vi "NewGrphWindow.vi"(8 "error in (no error)":errorcluster caption="entrée d'erreur (pas d'erreur)", 10 "CurvesIndx":i32[](array[numeric]), 11 "Interface en entrée":refnum<class "Interface.lvclass"> caption="DNL_LabVIEW Object in") -> (0 "error out":errorcluster caption="sortie d'erreur", 3 "Interface en sortie":refnum<class "Interface.lvclass"> caption="DNL_LabVIEW Object out")   [LabVIEW 2010, in "Interface.lvclass"]
uses:
  Interface.lvclass
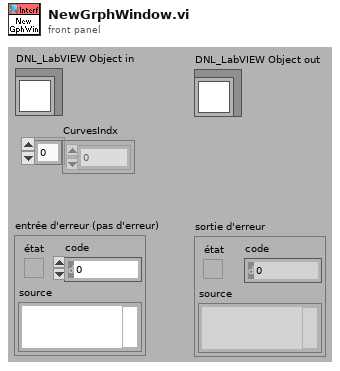
[diagram p1: front panel]
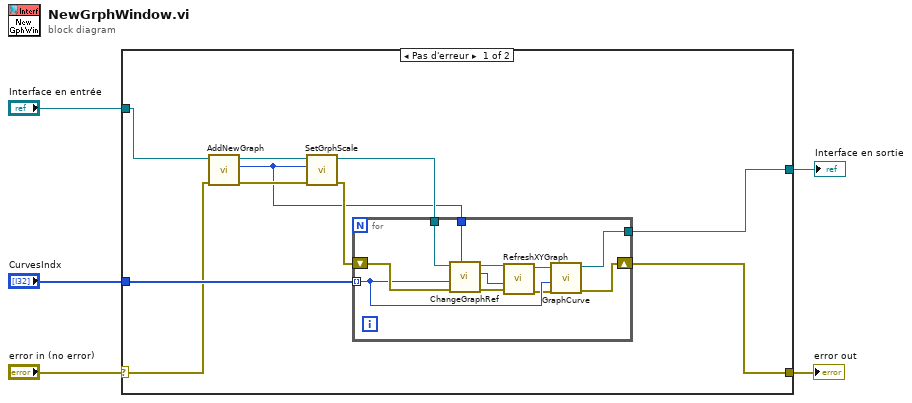
[diagram p0: block diagram]
diagram:
  n1 = case shown="Pas d'erreur" "error in (no error)" {
    selector: "error in (no error)" -> [w12 w28]
    tunnel: [w14 w28] -> w4
    tunnel: [w13 w27] -> w2
    tunnel: "Interface en entrée" -> [w11 w27]
    tunnel: "CurvesIndx" -> [w15 _]
    frame No Error {
      n2 = call "AddNewGraph.vi"("error in (no error)"=w12, "Interface en entrée"=w11) -> ("error out"=w8:errorcluster, "NewGraphInd"=w6:i32, "Interface en sortie"=w10:refnum<class "Interface.lvclass">)  [unwired: 7 in]
      n3 = call "SetGrphScale.vi"("error in (no error)"=w8, "GraphIndex"=w6, "Interface en entrée"=w10) -> ("error out"=w7:errorcluster, "Interface en sortie"=w9:refnum<class "Interface.lvclass">)  [unwired: 7 in]
      n4 = for {
        tunnel: w15 -> [w21] mode=indexing
        tunnel: w9 -> [w25]
        shift-right: [w24] -> w14
        shift-left: w7 -> [w26]
        tunnel: [w23] -> w13
        tunnel: w6 -> [w22]
        n5 = call "ChangeGraphRef.vi"("NewGraphIndex"=w22, "error in (no error)"=w26, "CurveIndex"=w21, "Interface en entrée"=w25) -> ("error out"=w17:errorcluster, "OldGraphIndex"=w16:i32, "Interface en sortie"=w18:refnum<class "Interface.lvclass">)  [unwired: 5 in]
        n6 = call "RefreshXYGraph.vi"("error in (no error)"=w17, "Graph Index"=w16, "Interface en entrée"=w18) -> ("error out"=w20:errorcluster, "Interface en sortie"=w19:refnum<class "Interface.lvclass">)  [unwired: 5 in, 2 out]
        n7 = call "GraphCurve.vi"("error in (no error)"=w20, "CurvIndex"=w21, "Interface en entrée"=w19) -> ("error out"=w24:errorcluster, "Interface en sortie"=w23:refnum<class "Interface.lvclass">)  [unwired: 7 in]
      }
    }
    frame Error {
    }
  }
  "error out" <- w4
  "Interface en sortie" <- w2
